vi "LIN weiter schalten und Fehlerbehandlung.vi"(0 "Anforderung in":bool, 1 "automatisch in":T3, 2 "TestRun":bool, 5 "Error in":bool, 7 "Gasteiler Type":T1 items=["LNI", "Analog-Display", "AVL GDU", "Horiba GDC", "HovaCal", "Horiba SGD 710C"], 9 "Referenzen Cluster":T2, 11 "error in (no error)":errorcluster caption="Fehler (Eingang, kein Fehler)", 12 "get Test Data":bool, 13 "running in":bool, 14 "Beendet":bool) -> (4 "Anforderung out":bool, 8 "Gasteiler Type out":T1 caption="Gasteiler Type" items=["LNI", "Analog-Display", "AVL GDU", "Horiba GDC", "HovaCal", "Horiba SGD 710C"], 15 "error out":errorcluster caption="Fehler (Ausgang)")   [LabVIEW 2020, in "Linearisierung v2.lvlib"]
uses:
  Linearisierung v2.lvlib
  Seiten/System Einstellungen V2/Konfig Gasflasche.ctl
  GasteilerType.ctl
  Visualisierungs Elemente/Button.ctl
  SpanEinstellungen/Aktion FGV SPAN Verriegelung.ctl
  SpanEinstellungen/Aktion FGV Spans abarbeiten.ctl
  SpanEinstellungen/SpanEinstellungen.lvlib
  Seiten/System Einstellungen V2/System Einstellungen V2.lvlib
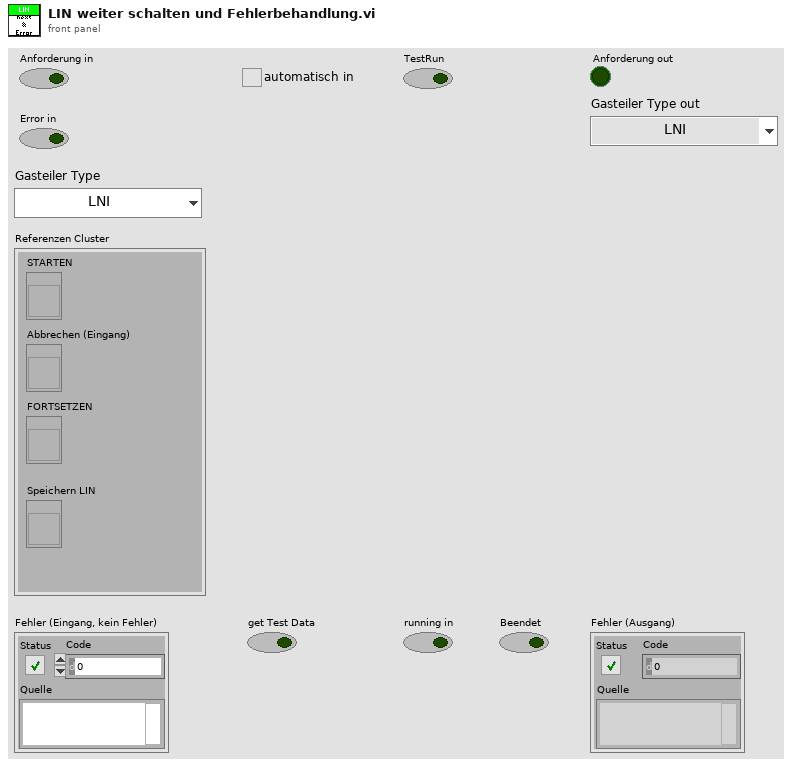
[diagram p1: front panel]
types:
  T1 = typedef "Linearisierung v2.lvlib/GasteilerType.ctl" = u16
  T2 = cluster{"STARTEN":refnum<vi>, "Abbrechen (Eingang)":refnum<vi>, "FORTSETZEN":refnum<vi>, "Speichern LIN":refnum<vi>}
  T3 = typedef "System Einstellungen V2.lvlib/Konfig Gasflasche.ctl" = bool
  T4 = typedef "Button.ctl" = bool
  T5 = enum8{"Enabled", "Disabled", "Disabled and Grayed Out"}
  T6 = typedef "Linearisierung v2.lvlib/SpanEinstellungen.lvlib/Aktion FGV Spans abarbeiten.ctl" = enum16{"lesen", "idle", "start", "next", "comp", "init", "running", "abort"}
  T7 = typedef "Linearisierung v2.lvlib/SpanEinstellungen.lvlib/Aktion FGV SPAN Verriegelung.ctl" = enum16{"lesen", "setrefs", "setcomp", "lock", "unlock", "Set Save EPA redirect", "Reset Save EPA redirect", "Set Postprocessing PDF", "Reset Postprocessing PDF", "Set Start Postprocessing PDF", "Reset Start Postprocessing PDF"}
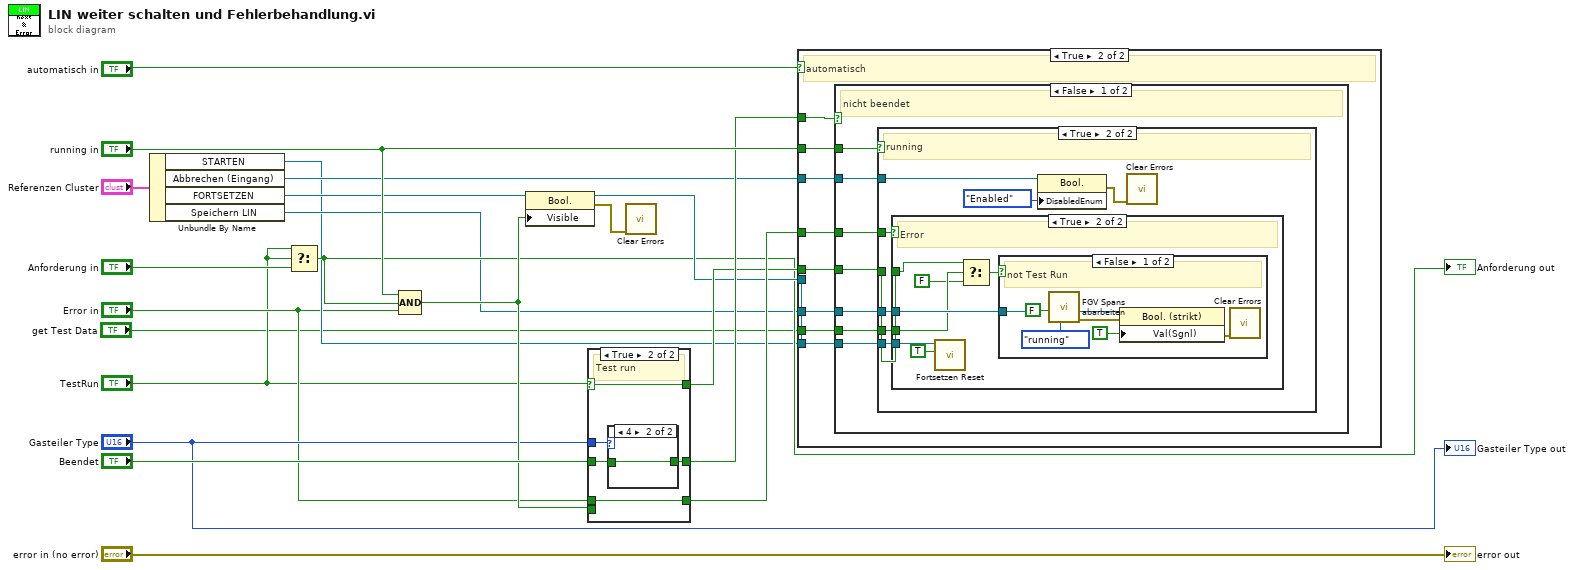
[diagram p0: block diagram]
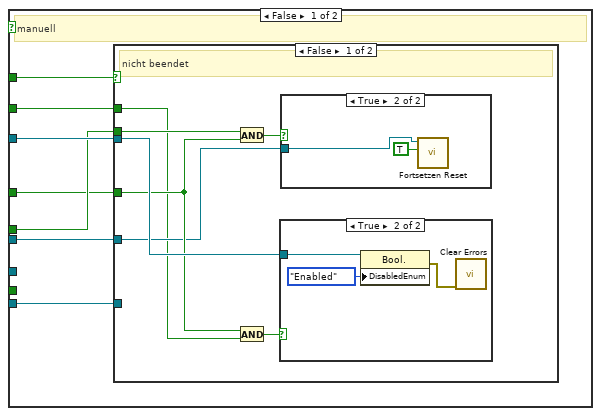
[diagram p4: hidden frame]
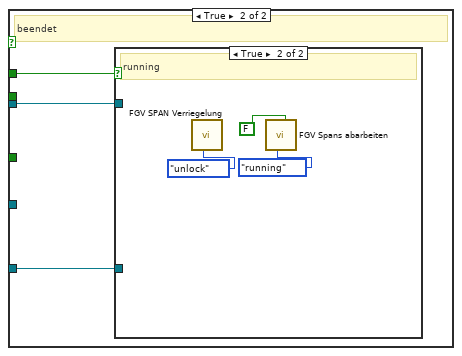
[diagram p7: hidden frame]
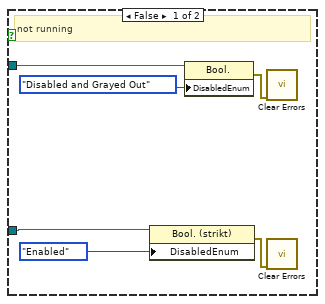
[diagram p8: hidden frame]
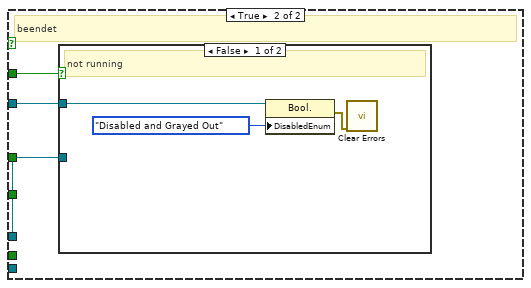
[diagram p12: hidden frame]
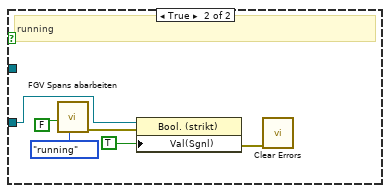
[diagram p13: hidden frame]
diagram:
  n1 = Unbundle By Name("Referenzen Cluster") -> ("STARTEN"=w5:refnum<vi>, "Abbrechen (Eingang)"=w6:refnum<vi>, "FORTSETZEN"=w7:refnum<vi>, "Speichern LIN"=w8:refnum<vi>)
  n2 = Select(t="TestRun", s="TestRun", f="Anforderung in") -> (s? t:f=w12:bool)
  "Anforderung out" <- w12
  n3 = Compound Arithmetic op=AND ("Mehrfacharithmetik")("running in", w12, "Error in") -> (w14:bool)
  n4 = property class="Bool."(reference=w7, "Visible"=w14) -> (reference out=w13:refnum<vi>, error out=w15:errorcluster)  [unwired: 1 in]
  n5 = case shown="True" "TestRun" {
    selector: "TestRun" -> [_ w24]
    tunnel: [w23 w26] -> w19
    tunnel: "Beendet" -> [w23 w27]
    tunnel: "Gasteiler Type" -> [_ w28]
    tunnel: "Error in" -> [_ w25]
    tunnel: [w22 w25] -> w20
    tunnel: w14 -> [w22 _]
    tunnel: [_ w24] -> w17
    frame False {
    }
    frame True {
      # "Test run"
      n6 = case shown="4" w28 {
        tunnel: w27 -> [w29 w30]
        tunnel: [w29 w30] -> w26
        frame 0, Default {
        }
        frame 4 {
        }
      }
    }
  }
  n7 = call <vilib>:"Clear Errors.vi"("error in (no error)"=w15) -> ()  [unwired: 5 in, 2 out]
  n8 = case shown="True" "automatisch in" {
    tunnel: w8 -> [_ w69]
    tunnel: w13 -> [w34 w68]
    tunnel: w19 -> [w37 w67]
    tunnel: "running in" -> [w33 w66]
    tunnel: w5 -> [w36 _]
    tunnel: w6 -> [w35 w63]
    tunnel: w17 -> [w32 w65]
    tunnel: w20 -> [w31 w64]
    tunnel: "get Test Data" -> [_ w62]
    frame False {
      # "manuell"
      n9 = case shown="False" w37 {
        tunnel: w35 -> [w44 w51]
        tunnel: w31 -> [w41 _]
        tunnel: w36 -> [_ w50]
        tunnel: w32 -> [w40 _]
        tunnel: w33 -> [w38 w52]
        tunnel: w34 -> [w39 _]
        frame False {
          # "nicht beendet"
          n10 = And(x=w40, y=w41) -> (x .and. y?=w42:bool)
          n11 = And(x=w41, y=w38) -> (x .and. y?=w43:bool)
          n12 = case shown="True" w43 {
            tunnel: w44 -> [_ w48]
            frame False {
            }
            frame True {
              n13 = property class="Bool."(reference=w48, "DisabledEnum"=T5."Enabled" ("Deaktiviert")) -> (error out=w49:errorcluster)  [unwired: 1 in, 1 out]
              n14 = call <vilib>:"Clear Errors.vi"("error in (no error)"=w49) -> ()  [unwired: 5 in, 2 out]
            }
          }
          n15 = case shown="True" w42 {
            tunnel: w39 -> [_ w45]
            frame False {
            }
            frame True {
              n16 = call "Fortsetzen Reset.vi"("FORTSETZEN"=T4 TRUE, "Referenz Boolesch (Eingang)"=w45) -> ()  [unwired: 10 in]
            }
          }
        }
        frame True {
          # "beendet"
          n17 = case shown="True" w52 {
            tunnel: w51 -> [w54 _]
            tunnel: w50 -> [w53 _]
            frame False {
              # "not running"
              n18 = property class="Bool. (strikt)"(reference=w53, "DisabledEnum"=T5."Enabled" ("Deaktiviert")) -> (error out=w57:errorcluster)  [unwired: 1 in, 1 out]
              n19 = property class="Bool."(reference=w54, "DisabledEnum"=T5."Disabled and Grayed Out" ("Deaktiviert")) -> (error out=w58:errorcluster)  [unwired: 1 in, 1 out]
              n20 = call <vilib>:"Clear Errors.vi"("error in (no error)"=w58) -> ()  [unwired: 5 in, 2 out]
              n21 = call <vilib>:"Clear Errors.vi"("error in (no error)"=w57) -> ()  [unwired: 5 in, 2 out]
            }
            frame True {
              # "running"
              n22 = call "FGV SPAN Verriegelung.vi"("aktion"=Aktion_FGV_SPAN_Verriegelung."unlock") -> ()  [unwired: 8 in, 3 out]
              n23 = call "FGV Spans abarbeiten.vi"("running"=FALSE, "Aktion"=Aktion_FGV_Spans_abarbeiten."running") -> ()  [unwired: 4 in, 6 out]
            }
          }
        }
      }
    }
    frame True {
      # "automatisch"
      n24 = case shown="False" w67 {
        tunnel: w69 -> [w76 w100]
        tunnel: w68 -> [w75 _]
        tunnel: w66 -> [w74 w98]
        tunnel: w65 -> [w73 _]
        tunnel: w64 -> [w72 _]
        tunnel: w63 -> [w71 w99]
        tunnel: w62 -> [w70 _]
        frame False {
          # "nicht beendet"
          n25 = case shown="True" w74 {
            tunnel: w76 -> [_ w83]
            tunnel: w75 -> [_ w82]
            tunnel: w73 -> [_ w81]
            tunnel: w72 -> [_ w80]
            tunnel: w71 -> [_ w79]
            tunnel: w70 -> [_ w77]
            frame False {
              # "not running"
            }
            frame True {
              # "running"
              n26 = case shown="True" w80 {
                tunnel: w82 -> [_ w90]
                tunnel: w83 -> [_ w89]
                tunnel: w81 -> [_ w87]
                tunnel: w77 -> [_ w88]
                frame False {
                }
                frame True {
                  # "Error"
                  n27 = call "Fortsetzen Reset.vi"("FORTSETZEN"=T4 TRUE, "Referenz Boolesch (Eingang)"=w90) -> ()  [unwired: 10 in]
                  n28 = Select(t=w87, s=w88, f=FALSE ("t")) -> (s? t:f=w86:bool)
                  n29 = case shown="False" w86 {
                    tunnel: w89 -> [w92 _]
                    frame False {
                      # "not Test Run"
                      n30 = call "FGV Spans abarbeiten.vi"("running"=FALSE, "Aktion"=Aktion_FGV_Spans_abarbeiten."running") -> ("error out"=w93:errorcluster)  [unwired: 4 in, 5 out]
                      n31 = property on="Eigenschaftsknoten" class="Bool. (strikt)"(reference=w92, error in=w93, "Val(Sgnl)"=T4 TRUE ("Wert (signalisierend)")) -> (error out=w96:errorcluster)  [unwired: 1 out]
                      n32 = call <vilib>:"Clear Errors.vi"("error in (no error)"=w96) -> ()  [unwired: 5 in, 2 out]
                    }
                    frame True {
                      # "Test Run"
                    }
                  }
                }
              }
              n33 = property class="Bool."(reference=w79, "DisabledEnum"=T5."Enabled" ("Deaktiviert")) -> (error out=w78:errorcluster)  [unwired: 1 in, 1 out]
              n34 = call <vilib>:"Clear Errors.vi"("error in (no error)"=w78) -> ()  [unwired: 5 in, 2 out]
            }
          }
        }
        frame True {
          # "beendet"
          n35 = case shown="False" w98 {
            tunnel: w100 -> [_ w104]
            tunnel: w99 -> [w102 _]
            frame False {
              # "not running"
              n36 = property class="Bool."(reference=w102, "DisabledEnum"=T5."Disabled and Grayed Out" ("Deaktiviert")) -> (error out=w101:errorcluster)  [unwired: 1 in, 1 out]
              n37 = call <vilib>:"Clear Errors.vi"("error in (no error)"=w101) -> ()  [unwired: 5 in, 2 out]
            }
            frame True {
              # "running"
              n38 = call "FGV Spans abarbeiten.vi"("running"=FALSE, "Aktion"=Aktion_FGV_Spans_abarbeiten."running") -> ("error out"=w105:errorcluster)  [unwired: 4 in, 5 out]
              n39 = property on="Eigenschaftsknoten" class="Bool. (strikt)"(reference=w104, error in=w105, "Val(Sgnl)"=T4 TRUE ("Wert (signalisierend)")) -> (error out=w108:errorcluster)  [unwired: 1 out]
              n40 = call <vilib>:"Clear Errors.vi"("error in (no error)"=w108) -> ()  [unwired: 5 in, 2 out]
            }
          }
        }
      }
    }
  }
  "Gasteiler Type out" <- "Gasteiler Type"
  "error out" <- "error in (no error)"
